vi "Configure Percent Deviation Calculation.vi"(6 "Use Input Signal as Reference Value (F: Disable)":bool, 8 "error in (no error)":errorcluster, 9 "Math Calculation (0.000000E+0)":dbl format="%.6e", 10 "Percent Target (1.000000E+0)":dbl=1.0 format="%.6e", 11 "VISA resource name":refnum<visa-resource-name>) -> (0 "error out":errorcluster, 3 "VISA resource name out":refnum<visa-resource-name>)   [LabVIEW 2016, in "Keithley 6517.lvlib"]
doc: "Configures the target value for the percent calculation and set the reference value for ratio, deviation, and percent deviation calculation."
uses:
  <instrlib>/Keithley 6517/Keithley 6517.lvlib
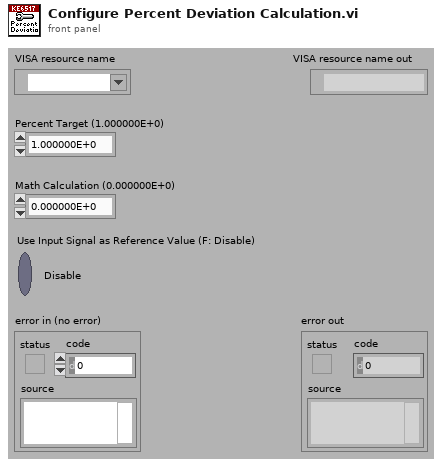
[diagram p1: front panel]
types:
  T1 = typedef "Keithley 6517.lvlib/Extended User Data.ctl" = cluster{"Instrument Model":i32}
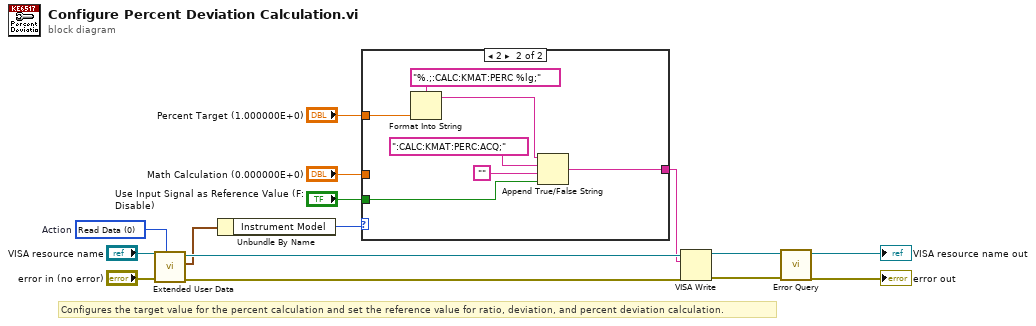
[diagram p0: block diagram]
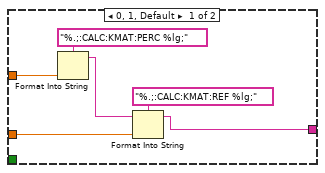
[diagram p2: hidden frame]
diagram:
  w5 = u16 0 items=["Read Data", "Write Data", "Clear Data", "Clear ALL Data"]  # Action
  # "Configures the target value for the percent calculation and set the reference value for ratio, deviation, and percent deviation calculation."
  n1 = call <instrlib>:"Extended User Data.vi"("Action (0: Read Data)"=w5, "error in (no error)"="error in (no error)", "VISA resource name"="VISA resource name") -> ("error out"=w7:errorcluster, "User Data Out"=w4:T1, "VISA resource name out"=w6:refnum<visa-resource-name>)  [unwired: 6 in]
  n2 = Unbundle By Name(w4) -> ("Instrument Model"=w3:i32)
  n3 = case shown="2" w3 {
    tunnel: "Percent Target (1.000000E+0)" -> [w20 w27]
    tunnel: "Math Calculation (0.000000E+0)" -> [w17 _]
    tunnel: "Use Input Signal as Reference Value (F: Disable)" -> [_ w23]
    tunnel: [w16 w22] -> w1
    frame 0, 1, Default {
      n4 = Format Into String(format string="%.;:CALC:KMAT:PERC %lg;", w20) -> (resulting string=w19:string)  [unwired: 2 in, 1 out]
      n5 = Format Into String(format string="%.;:CALC:KMAT:REF %lg;", initial string=w19, w17) -> (resulting string=w16:string)  [unwired: 1 in, 1 out]
    }
    frame 2 {
      n6 = Format Into String(format string="%.;:CALC:KMAT:PERC %lg;", w27) -> (resulting string=w26:string)  [unwired: 2 in, 1 out]
      n7 = Append True/False String(1:w23, 2:"", 3:":CALC:KMAT:PERC:ACQ;" ("true string"), 4:w26) -> (0:w22:string)
    }
  }
  n8 = VISA Write(VISA resource name=w6, write buffer=w1, error in (no error)=w7) -> (VISA resource name out=w13:refnum<visa-resource-name>, error out=w12:errorcluster)  [unwired: 1 out]
  n9 = call <instrlib>:"Error Query.vi"("error in (no error)"=w12, "VISA resource name"=w13) -> ("error out"=→"error out":errorcluster, "VISA resource name out"=→"VISA resource name out":refnum<visa-resource-name>)  [unwired: 6 in, 2 out]
